vi "Convert from String.vi"(8 "error in (no error)":errorcluster, 9 "data type":variant, 10 "String":string) -> (0 "error out":errorcluster, 2 "data":variant)   [LabVIEW 2023, in "uData.lvlib" / "uData.lvclass"]
doc: "Convert incoming data type to string."
uses:
  uData.lvclass
  uConvertible.lvclass
  <vilib>/Utility/error.llb/Error Cluster From Error Code.vi
  <vilib>/ErrorRing/Error Ring.xnode
  uData.lvclass/uData.ctl
  <vilib>/Utility/Data Type/NI_Data Type.lvlib
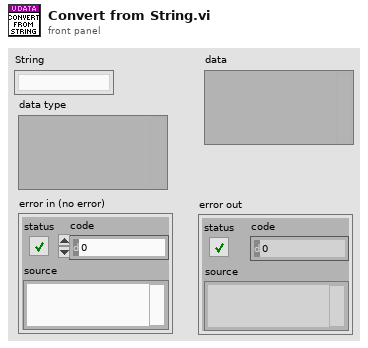
[diagram p1: front panel]
types:
  T1 = typedef "NI_Data Type.lvlib/Data Type.ctl" = enum8{"Invalid Type", "Void", "I8", "I16", "I32", "I64", "U8", "U16", "U32", "U64", "Single Float", "Double Float", "Extended Float", "Single Complex", "Double Complex", "Extended Complex", "Enum U8", "Enum U16", "Enum U32", "Enum U64", "Single Float With Unit", "Double Float With Unit", "Extended Float With Unit", "Single Complex with Unit", "Double Complex with Unit", "Extended Complex with Unit", "Boolean", "String", "Path", "Picture", "Tag", "Array", "Cluster", "Variant", "LV Variant", "Waveform", "Timestamp", "Digital Waveform", "Digital Data", "ExpressData", "Refnum", "External Data", "VI", "Poly VI", "LabVIEW Class Instance", "Fixed Point", "Set Collection", "Map Collection"}
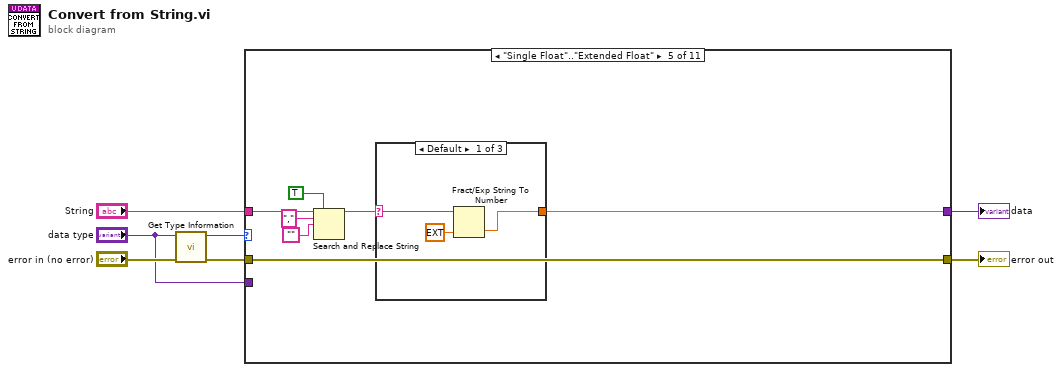
[diagram p0: block diagram]
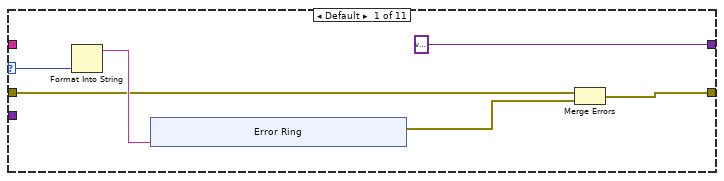
[diagram p2: hidden frame]
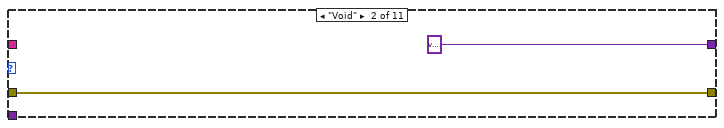
[diagram p3: hidden frame]
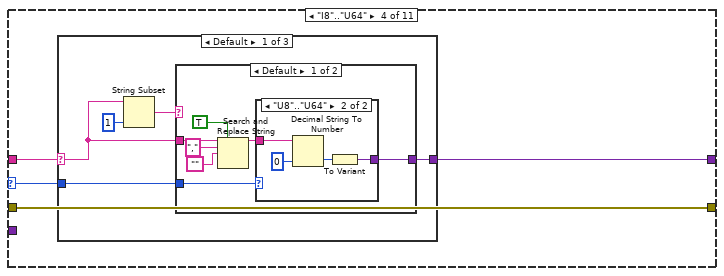
[diagram p5: hidden frame]
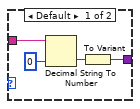
[diagram p6: hidden frame]
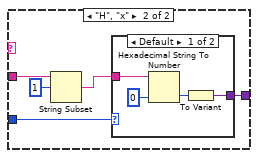
[diagram p7: hidden frame]
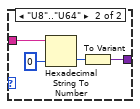
[diagram p8: hidden frame]
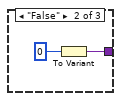
[diagram p9: hidden frame]
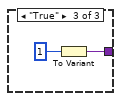
[diagram p10: hidden frame]
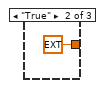
[diagram p11: hidden frame]
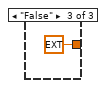
[diagram p12: hidden frame]
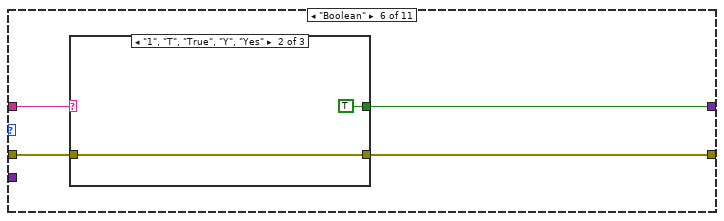
[diagram p13: hidden frame]
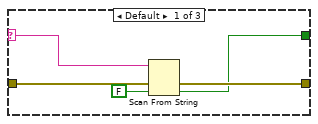
[diagram p14: hidden frame]
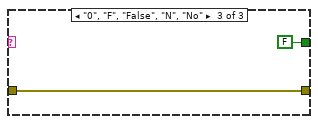
[diagram p15: hidden frame]
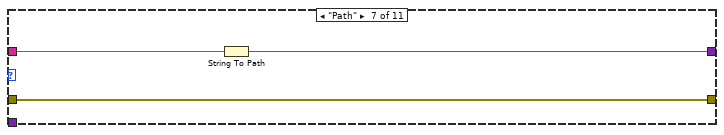
[diagram p16: hidden frame]
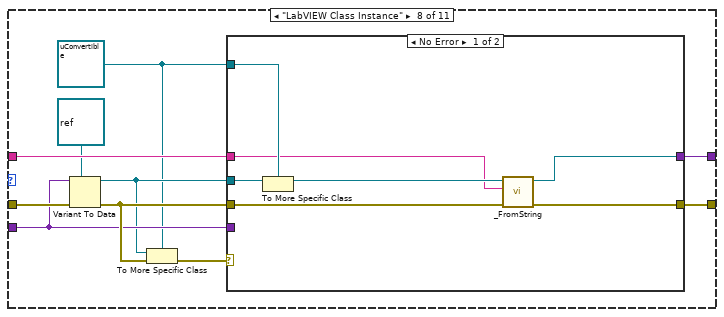
[diagram p17: hidden frame]
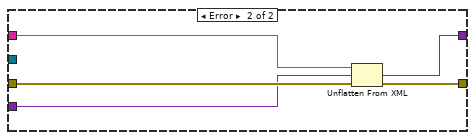
[diagram p18: hidden frame]
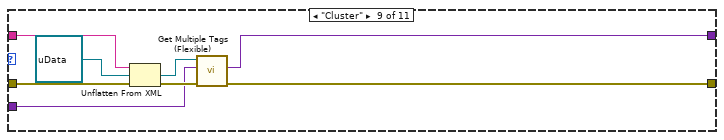
[diagram p19: hidden frame]
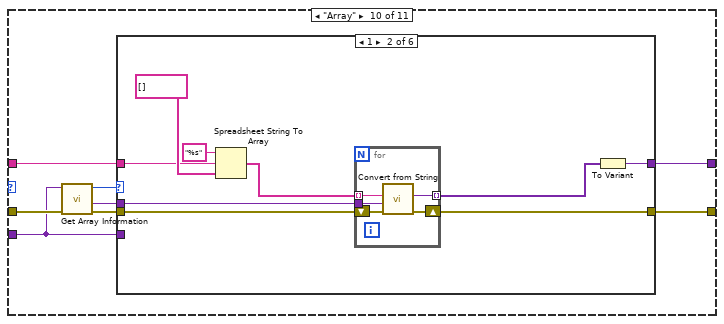
[diagram p20: hidden frame]
diagram:
  n1 = call <vilib>:"Get Type Information.vi"("error in (no error)"="error in (no error)", "variant"="data type") -> ("error out"=w4:errorcluster, "type"=w6:T1)  [unwired: 5 in, 3 out]
  n2 = case shown="\"Single Float\"..\"Extended Float\"" w6 {
    selector: w6 -> [w13 _ _ w25 _ _ _ _ _ _ _]
    tunnel: [w9 w22 w24 w28 w72 w80 w91 w103 w117 w128 w258] -> w5
    tunnel: w4 -> [w8 w22 w24 w28 w72 w81 w91 w100 w123 w129 w258]
    tunnel: "String" -> [_ _ w23 w26 w66 w78 w93 w102 w122 w127 _]
    tunnel: [variant variant ("String") w23 w27 w71 w79 w92 w101 w116 w126 w257] -> w2
    tunnel: "data type" -> [_ _ _ _ _ _ _ w98 w119 w125 w257]
    frame Default {
      n3 = Format Into String(w13) -> (resulting string=w12:string)  [unwired: 3 in, 1 out]
      n4 = xnode "Error Ring"("parameter 0"=w12) -> ("error out"=w10:errorcluster)
      n5 = Merge Errors(w8, w10) -> (w9:errorcluster)
    }
    frame "Void" {
    }
    frame "String" {
    }
    frame "I8".."U64" {
      n6 = case shown="Default" w26 {
        selector: w26 -> [w30 _ _]
        tunnel: [w33 w63 w65] -> w27
        tunnel: w25 -> [w29 _ _]
        frame Default {
          n7 = String Subset(string=w30, length (rest)=1 ("length (rest)")) -> (substring=w31:string)  [unwired: 1 in]
          n8 = case shown="Default" w31 {
            tunnel: [w39 w49] -> w33
            tunnel: w30 -> [w37 w53]
            tunnel: w29 -> [w40 w50]
            frame Default {
              n9 = Search and Replace String(replace all?=TRUE ("replace all? (F)"), input string=w37, search string=",", replace string="") -> (result string=w38:string)  [unwired: 4 in, 3 out]
              n10 = case shown="\"U8\"..\"U64\"" w40 {
                tunnel: [w41 w45] -> w39
                tunnel: w38 -> [w42 w46]
                frame Default {
                  n11 = Decimal String To Number(string=w42, default (0L)=i64 0 ("default (0 U32)")) -> (number=w44:i64)  [unwired: 1 in, 1 out]
                  n12 = To Variant(anything=w44) -> (Variant=w41:variant)
                }
                frame "U8".."U64" {
                  n13 = Decimal String To Number(string=w46, default (0L)=u64 0 ("default (0 U32)")) -> (number=w48:u64)  [unwired: 1 in, 1 out]
                  n14 = To Variant(anything=w48) -> (Variant=w45:variant)
                }
              }
            }
            frame "H", "x" {
              n15 = String Subset(string=w53, offset (0)=1) -> (substring=w52:string)  [unwired: 1 in]
              n16 = case shown="Default" w50 {
                tunnel: [w54 w58] -> w49
                tunnel: w52 -> [w55 w59]
                frame Default {
                  n17 = Hexadecimal String To Number(string=w55, default (0uL)=i64 0 ("default (0 U32)")) -> (number=w57:i64)  [unwired: 1 in, 1 out]
                  n18 = To Variant(anything=w57) -> (Variant=w54:variant)
                }
                frame "U8".."U64" {
                  n19 = Hexadecimal String To Number(string=w59, default (0uL)=u64 0 ("default (0 U32)")) -> (number=w61:u64)  [unwired: 1 in, 1 out]
                  n20 = To Variant(anything=w61) -> (Variant=w58:variant)
                }
              }
            }
          }
        }
        frame "False" {
          n21 = To Variant(anything=0) -> (Variant=w63:variant)
        }
        frame "True" {
          n22 = To Variant(anything=1) -> (Variant=w65:variant)
        }
      }
    }
    frame "Single Float".."Extended Float" {
      n23 = Search and Replace String(replace all?=TRUE ("replace all? (F)"), input string=w66, search string=",", replace string="") -> (result string=w67:string)  [unwired: 4 in, 3 out]
      n24 = case shown="Default" w67 {
        selector: w67 -> [w73 _ _]
        tunnel: [w75 ext 1.0 ext 0.0] -> w71
        frame Default {
          n25 = Fract/Exp String To Number(string=w73, default (0 dbl)=ext 0.0 ("default (0 DBL)")) -> (number=w75:ext)  [unwired: 2 in, 1 out]
        }
        frame "True" {
        }
        frame "False" {
        }
      }
    }
    frame "Boolean" {
      n26 = case shown="\"1\", \"T\", \"True\", \"Y\", \"Yes\"" w78 {
        selector: w78 -> [w82 _ _]
        tunnel: w81 -> [w85 w87 w89]
        tunnel: [w84 w87 w89] -> w80
        tunnel: [w83 TRUE FALSE] -> w79
        frame Default {
          n27 = Scan From String(input string=w82, error in=w85, default 1=FALSE) -> (error out=w84:errorcluster, output 1=w83:bool)  [unwired: 2 in, 2 out]
        }
        frame "1", "T", "True", "Y", "Yes" {
        }
        frame "0", "F", "False", "N", "No" {
        }
      }
    }
    frame "Path" {
      n28 = String To Path(string=w93) -> (path=w92:path)
    }
    frame "LabVIEW Class Instance" {
      w94 = refnum<class "uConvertible.lvclass"> refnum ("uData.lvlib:uConvertible.lvclass")
      n29 = Variant To Data(error in=w100, type=refnum<class> refnum ("LabVIEW Object"), Variant=w98) -> (data=w95:refnum<class>, error out=w99:errorcluster)
      n30 = To More Specific Class(target class=w94, reference=w95, error in=w99) -> (error out=w97:errorcluster)  [unwired: 1 out]
      n31 = case shown="No Error" w97 {
        tunnel: [w106 w115] -> w103
        tunnel: w102 -> [w105 w114]
        tunnel: [w104 w113] -> w101
        tunnel: w99 -> [w108 w112]
        tunnel: w98 -> [_ w111]
        tunnel: w94 -> [w110 _]
        tunnel: w95 -> [w109 _]
        frame No Error {
          n32 = To More Specific Class(target class=w110, reference=w109) -> (specific class reference=w107:refnum<class "uConvertible.lvclass">)  [unwired: 1 in, 1 out]
          n33 = call-dynamic "_FromString.vi"("error in (no error)"=w108, "FromString"=w105, "uConvertible in"=w107) -> ("error out"=w106:errorcluster, "uConvertible out"=w104:refnum<class "uConvertible.lvclass">)  [unwired: 7 in]
        }
        frame Error {
          n34 = Unflatten From XML(xml string=w114, type=w111, error in (no error)=w112) -> (value=w113:variant, error out=w115:errorcluster)
        }
      }
    }
    frame "Cluster" {
      n35 = Unflatten From XML(xml string=w122, type=refnum<class "uData.lvclass"> refnum ("iData in"), error in (no error)=w123) -> (value=w118:refnum<class "uData.lvclass">, error out=w120:errorcluster)
      n36 = call "Get Multiple Tags (Flexible).vi"("error in (no error)"=w120, "Cluster"=w119, "uData in"=w118) -> ("error out"=w117:errorcluster, "data"=w116:variant)  [unwired: 4 in, 3 out]
    }
    frame "Array" {
      n37 = call <vilib>:"Get Array Information.vi"("error in (no error)"=w129, "variant"=w125) -> ("error out"=w131:errorcluster, "array element data type"=w124:variant, "number of dimensions"=w130:i32)  [unwired: 6 in, 1 out]
      n38 = case shown="1" w130 {
        tunnel: w131 -> [w134 w144 w158 w177 w201 w230]
        tunnel: [w133 w145 w159 w178 w202 w231] -> w128
        tunnel: w127 -> [_ w137 w152 w171 w195 w224]
        tunnel: [variant ("Variant") w140 w154 w173 w197 w226] -> w126
        tunnel: w125 -> [_ _ _ _ _ _]
        tunnel: w124 -> [_ w139 w153 w172 w196 w225]
        frame Default {
          n39 = xnode "Error Ring"() -> ("error out"=w132:errorcluster)
          n40 = Merge Errors(w134, w132) -> (w133:errorcluster)
        }
        frame 1 {
          n41 = Spreadsheet String To Array(format string="%s" ("spreadsheet string"), spreadsheet string=w137, array type (2D Dbl)=string[] [] ("type")) -> (array=w142:string[])  [unwired: 1 in]
          n42 = for {
            shift-right: [w149] -> w145
            shift-left: w144 -> [w150]
            tunnel: [w148] -> w141 mode=indexing
            tunnel: w142 -> [w147] mode=indexing
            tunnel: w139 -> [w146]
            n43 = call "Convert from String.vi"("error in (no error)"=w150, "data type"=w146, "String"=w147) -> ("error out"=w149:errorcluster, "data"=w148:variant)  [unwired: 7 in]
          }
          n44 = To Variant(anything=w141) -> (Variant=w140:variant)
        }
        frame 2 {
          n45 = Spreadsheet String To Array(format string="%s" ("spreadsheet string"), spreadsheet string=w152, array type (2D Dbl)=string[][] [] ("type")) -> (array=w156:string[][])  [unwired: 1 in]
          n46 = for {
            tunnel: w156 -> [w162] mode=indexing
            tunnel: [w161] -> w155 mode=indexing
            shift-right: [w164] -> w159
            shift-left: w158 -> [w163]
            tunnel: w153 -> [w160]
            n47 = for {
              shift-right: [w168] -> w164
              shift-left: w163 -> [w169]
              tunnel: [w167] -> w161 mode=indexing
              tunnel: w162 -> [w166] mode=indexing
              tunnel: w160 -> [w165]
              n48 = call "Convert from String.vi"("error in (no error)"=w169, "data type"=w165, "String"=w166) -> ("error out"=w168:errorcluster, "data"=w167:variant)  [unwired: 7 in]
            }
          }
          n49 = To Variant(anything=w155) -> (Variant=w154:variant)
        }
        frame 3 {
          n50 = Spreadsheet String To Array(format string="%s" ("spreadsheet string"), spreadsheet string=w171, array type (2D Dbl)=string[][][] [] ("type")) -> (array=w175:string[][][])  [unwired: 1 in]
          n51 = for {
            tunnel: w175 -> [w181] mode=indexing
            tunnel: [w180] -> w174 mode=indexing
            shift-right: [w183] -> w178
            shift-left: w177 -> [w182]
            tunnel: w172 -> [w179]
            n52 = for {
              tunnel: w181 -> [w186] mode=indexing
              tunnel: [w185] -> w180 mode=indexing
              shift-right: [w188] -> w183
              shift-left: w182 -> [w187]
              tunnel: w179 -> [w184]
              n53 = for {
                shift-right: [w192] -> w188
                shift-left: w187 -> [w193]
                tunnel: [w191] -> w185 mode=indexing
                tunnel: w186 -> [w190] mode=indexing
                tunnel: w184 -> [w189]
                n54 = call "Convert from String.vi"("error in (no error)"=w193, "data type"=w189, "String"=w190) -> ("error out"=w192:errorcluster, "data"=w191:variant)  [unwired: 7 in]
              }
            }
          }
          n55 = To Variant(anything=w174) -> (Variant=w173:variant)
        }
        frame 4 {
          n56 = Spreadsheet String To Array(format string="%s" ("spreadsheet string"), spreadsheet string=w195, array type (2D Dbl)=string[][][][] [] ("type")) -> (array=w199:string[][][][])  [unwired: 1 in]
          n57 = for {
            tunnel: w199 -> [w205] mode=indexing
            tunnel: [w204] -> w198 mode=indexing
            shift-right: [w207] -> w202
            shift-left: w201 -> [w206]
            tunnel: w196 -> [w203]
            n58 = for {
              tunnel: w205 -> [w210] mode=indexing
              tunnel: [w209] -> w204 mode=indexing
              shift-right: [w212] -> w207
              shift-left: w206 -> [w211]
              tunnel: w203 -> [w208]
              n59 = for {
                tunnel: w210 -> [w215] mode=indexing
                tunnel: [w214] -> w209 mode=indexing
                shift-right: [w217] -> w212
                shift-left: w211 -> [w216]
                tunnel: w208 -> [w213]
                n60 = for {
                  shift-right: [w221] -> w217
                  shift-left: w216 -> [w222]
                  tunnel: [w220] -> w214 mode=indexing
                  tunnel: w215 -> [w219] mode=indexing
                  tunnel: w213 -> [w218]
                  n61 = call "Convert from String.vi"("error in (no error)"=w222, "data type"=w218, "String"=w219) -> ("error out"=w221:errorcluster, "data"=w220:variant)  [unwired: 7 in]
                }
              }
            }
          }
          n62 = To Variant(anything=w198) -> (Variant=w197:variant)
        }
        frame 5 {
          n63 = Spreadsheet String To Array(format string="%s", spreadsheet string=w224, array type (2D Dbl)=string[][][][][] [] ("type")) -> (array=w228:string[][][][][])  [unwired: 1 in]
          n64 = for {
            tunnel: w228 -> [w234] mode=indexing
            tunnel: [w233] -> w227 mode=indexing
            shift-right: [w236] -> w231
            shift-left: w230 -> [w235]
            tunnel: w225 -> [w232]
            n65 = for {
              tunnel: w234 -> [w239] mode=indexing
              tunnel: [w238] -> w233 mode=indexing
              shift-right: [w241] -> w236
              shift-left: w235 -> [w240]
              tunnel: w232 -> [w237]
              n66 = for {
                tunnel: w239 -> [w244] mode=indexing
                tunnel: [w243] -> w238 mode=indexing
                shift-right: [w246] -> w241
                shift-left: w240 -> [w245]
                tunnel: w237 -> [w242]
                n67 = for {
                  tunnel: w244 -> [w249] mode=indexing
                  tunnel: [w248] -> w243 mode=indexing
                  shift-right: [w251] -> w246
                  shift-left: w245 -> [w250]
                  tunnel: w242 -> [w247]
                  n68 = for {
                    shift-right: [w255] -> w251
                    shift-left: w250 -> [w256]
                    tunnel: [w254] -> w248 mode=indexing
                    tunnel: w249 -> [w253] mode=indexing
                    tunnel: w247 -> [w252]
                    n69 = call "Convert from String.vi"("error in (no error)"=w256, "data type"=w252, "String"=w253) -> ("error out"=w255:errorcluster, "data"=w254:variant)  [unwired: 7 in]
                  }
                }
              }
            }
          }
          n70 = To Variant(anything=w227) -> (Variant=w226:variant)
        }
      }
    }
    frame "Enum U8".."Enum U64" {
      # "#RESERVED for future implementation"
    }
  }
  "data" <- w2
  "error out" <- w5
